vi "Console_SaveFile.vi"(8 "Path":path, 9 "Code":string, 11 "Queue in":refnum<queue>) -> ()   [LabVIEW 2022 SP3]
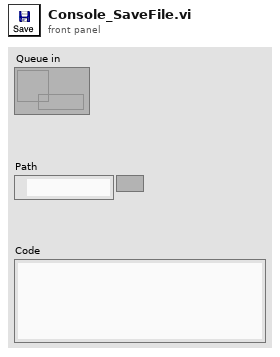
[diagram p1: front panel]
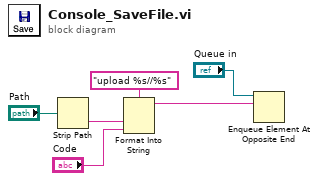
[diagram p0: block diagram]
diagram:
  n1 = Strip Path(path="Path") -> (name=w3:string)  [unwired: 1 out]
  n2 = Format Into String(format string="upload %s//%s", w3, "Code") -> (resulting string=w6:string)  [unwired: 2 in, 1 out]
  n3 = Enqueue Element At Opposite End(queue="Queue in", element=w6) -> ()  [unwired: 2 in, 3 out]
